vi "Save Profile (uSMC).vi"(8 "error in (no error)":errorcluster, 9 "SMIndex":i32, 10 "Profile path":path, 11 "Visa array in":refnum<visa-resource-name>[](array[refnum])) -> (0 "error out":errorcluster, 2 "Path (dup)":path, 3 "Visa array out":refnum<visa-resource-name>[](array[refnum]))   [LabVIEW 2010, in "SignalWriterMH110203USBStepperMotor.lvclass"]
uses:
  SignalWriterMH110203USBStepperMotor.lvclass
  class_data.vi
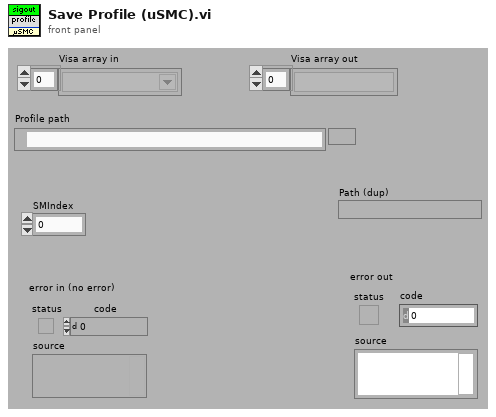
[diagram p1: front panel]
types:
  T1 = enum16{"open", "open or create", "create or replace", "create", "open (read only)"}
  T2 = typedef "SignalWriterMH110203USBStepperMotor.lvclass/Set Parameters (uSMC).ctl" = cluster{"Acceleration Time":u8, "Deceleration Time":u8, "Reduce Current Timeout":u16, "Buttons Timeout 1":u16, "Buttons Timeout 2":u16, "Buttons Timeout 3":u16, "Buttons Timeout 4":u16, "Buttons Timeout Reset":u16, "Buttons Timeout DblClick":u16, "Reset Speed":u16, "Buttons Speed 1":u16, "Buttons Speed 2":u16, "Buttons Speed 3":u16, "Buttons Speed 4":u16, "Max Backlash":u16, "Start Pos":i32, "RTdelta":u16, "RTMinError":u16, "Maximum Temperature":u16, "Sync Duration":u8, "Backlash Speed":u16, "EncVSCP":u8, "Steps Per Revolution":i32, "Encoder Pulses Per Rev-on":i32}
  T3 = typedef "SignalWriterMH110203USBStepperMotor.lvclass/GoTo Control (uSMC).ctl" = cluster{"Step motor ID":string, "SMname":string, "Backlash":u16, "wait for input sygnal to start":bool, "use slow start/stop":bool, "units name":string, "Maximum speed":dbl, "speed":dbl, "step":u8, "point 1 ticks":i32, "point 2 ticks":i32, "point 1 units":dbl, "point 2 units":dbl, "Limit Switch standoff":dbl, "Zero Value":dbl, "Destination Position":dbl, "force backlash":bool, "power off when stop":bool, "POff delay":dbl, "positioner name":string, "R, Ohm":dbl, "I, mA":dbl, "Positioner's Type":u16, "Reset Direction":bool, "Manufacturer":string, "Model":string, "Scheme":string, "FirmwareVer":string}
  T4 = cluster{"Cur Pos Units":dbl, "Set Cur Pos units":dbl, "Lo Limit Units":dbl, "Hi Limit Units":dbl, "Cur Pos Ticks":i32, "Set Cur Pos ticks":i32, "Lo Limit Ticks":i32, "Hi Limit Ticks":i32, "Minimal Value":dbl, "Maximal Value":dbl}[]
  T5 = typedef "SignalWriterMH110203USBStepperMotor.lvclass/Mode Control (uSMC).ctl" = cluster{"Turn Buttons Off":bool, "Reduce Current":bool, "Power Off and Make a Whole Step":bool, "Emergency Power Off":bool, "Limit Switch 1 True State":bool, "Limit Switch 2 True State":bool, "Rotary Transducer TRUE State":bool, "Swap Limit Switches":bool, "Limit Switch 1 Operation Enabled":bool, "Limit Switch 2 Operation Enabled":bool, "Rotary Transducer Operation Enabled":bool, "Rotary Transducer Operation Select":bool, "Button 1 True State":bool, "Button 2 True State":bool, "Swap Buttons":bool, "Reset Rotary Transducer Check Positions":bool, "Output Syncronization Enabled":bool, "Reset Output Sync Count":bool, "Sync Operation":bool, "Sync Count":u32, "Power":bool, "Invert Sync Polarity":bool, "Use Encoder":bool, "Invert Encoder Direction":bool, "Reset Encoder To 0":bool, "Reset SM Enc Pos to Enc Pos":bool}
  T6 = cluster{"Cur Pos Units":dbl, "Set Cur Pos units":dbl, "Lo Limit Units":dbl, "Hi Limit Units":dbl, "Cur Pos Ticks":i32, "Set Cur Pos ticks":i32, "Lo Limit Ticks":i32, "Hi Limit Ticks":i32, "Minimal Value":dbl, "Maximal Value":dbl}
  T7 = cluster{"Mode Defalults":T5, "Parameters Defalut":T2, "Position Default":cluster{"Cur Pos Units":dbl, "Set Cur Pos units":dbl, "Lo Limit Units":dbl, "Hi Limit Units":dbl, "Cur Pos Ticks":i32, "Set Cur Pos ticks":i32, "Lo Limit Ticks":i32, "Hi Limit Ticks":i32, "Minimal Value":dbl, "Maximal Value":dbl}, "StartPlus Default":T3}
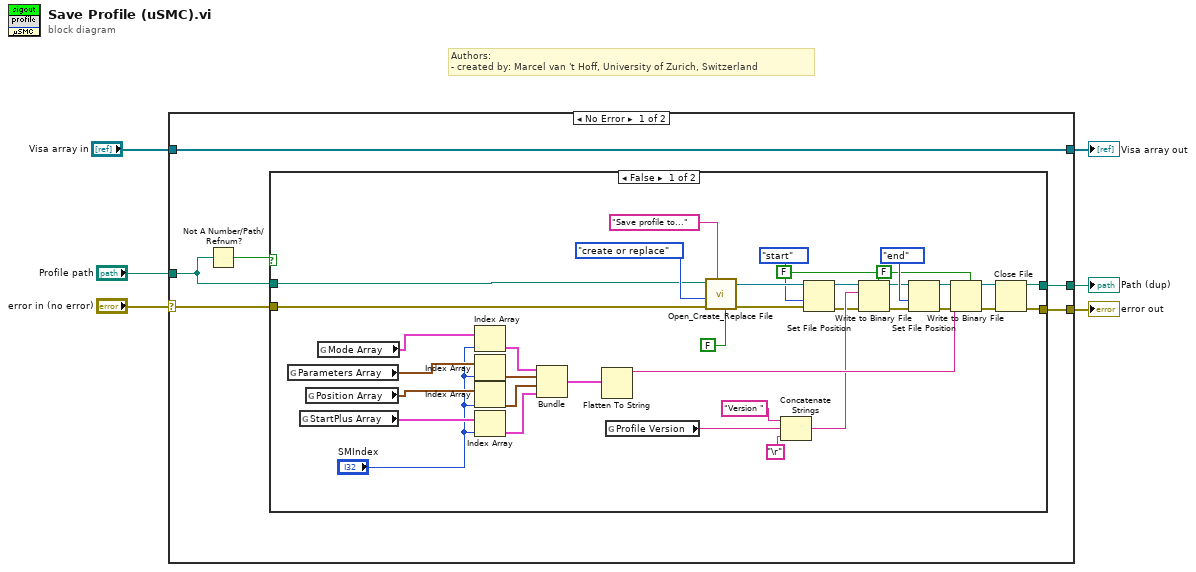
[diagram p0: block diagram]
diagram:
  # "Authors: \n- created by: Marcel van 't Hoff, University of Zurich, Switzerland"
  n1 = case shown="No Error" "error in (no error)" {
    selector: "error in (no error)" -> [w8 w52]
    tunnel: [w12 w52] -> w6
    tunnel: [w11 w51] -> w5
    tunnel: "Profile path" -> [w10 w51]
    tunnel: [w7 w53] -> w1
    tunnel: "Visa array in" -> [w7 w53]
    frame No Error {
      n2 = Not A Number/Path/Refnum?(number/path/refnum=w10) -> (NaN/Path/Refnum?=w9:bool)
      n3 = case shown="False" w9 {
        tunnel: w8 -> [w47 w49]
        tunnel: [w30 w49] -> w12
        tunnel: [w22 w50] -> w11
        tunnel: w10 -> [w19 w50]
        frame False {
          n4 = global read "class_data.vi" "Parameters Array"() -> (w33:T2[])
          n5 = global read "class_data.vi" "StartPlus Array"() -> (w31:T3[])
          n6 = global read "class_data.vi" "Position Array"() -> (w32:T4)
          n7 = global read "class_data.vi" "Mode Array"() -> (w34:T5[])
          n8 = Index Array(array=w34, index="SMIndex") -> (element=w43:T5)
          n9 = Index Array(array=w33, index="SMIndex") -> (element=w42:T2)
          n10 = Index Array(array=w32, index="SMIndex") -> (element=w41:T6)
          n11 = Index Array(array=w31, index="SMIndex") -> (element=w39:T3)
          n12 = Bundle("Mode Defalults"=w43, "Parameters Defalut"=w42, "Position Default"=w41, "StartPlus Default"=w39) -> (w40:T7)  [unwired: 1 in]
          n13 = Flatten To String(anything=w40) -> (data string=w44:string)  [unwired: 3 in, 2 out]
          n14 = global read "class_data.vi" "Profile Version"() -> (w21:string)
          n15 = call <vilib>:"Open_Create_Replace File.vi"("advisory dialog? (display:T)"=FALSE, "prompt"="Save profile to...", "error in (no error)"=w47, "function (open:0)"=T1."create or replace", "file path"=w19) -> ("error out"=w29:errorcluster, "refnum"=w26:refnum<file>)  [unwired: 3 in, 2 out]
          n16 = Concatenate Strings("Version " ("string"), w21, "\r") -> (w24:string)
          n17 = Set File Position(refnum=w26, from (0:start)=enum16{"start", "end", "current"}."start" ("pos mode (0:2)"), error in=w29) -> (refnum out=w18:refnum<file>, error out=w17:errorcluster)  [unwired: 1 in]
          n18 = Write to Binary File(file (use dialog)=w18, data=w24, error in=w17, 5:FALSE ("prepend array or string size? (T)")) -> (refnum out=w27:refnum<file>, error out=w28:errorcluster)  [unwired: 2 in, 1 out]
          n19 = Set File Position(refnum=w27, from (0:start)=enum16{"start", "end", "current"}."end" ("pos mode (0:2)"), error in=w28) -> (refnum out=w15:refnum<file>, error out=w14:errorcluster)  [unwired: 1 in]
          n20 = Write to Binary File(file (use dialog)=w15, data=w44, error in=w14, 5:FALSE ("prepend array or string size? (T)")) -> (refnum out=w38:refnum<file>, error out=w37:errorcluster)  [unwired: 2 in, 1 out]
          n21 = Close File(refnum=w38, error in=w37) -> (path=w22:path, error out=w30:errorcluster)
        }
        frame True {
        }
      }
    }
    frame Error {
    }
  }
  "error out" <- w6
  "Path (dup)" <- w5
  "Visa array out" <- w1
